vi "getValue.vi"(8 "error in (no error)":errorcluster, 11 "tBSONString in":refnum<class "tBSONString.lvclass">) -> (0 "error out":errorcluster, 2 "String":string, 3 "tBSONString out":refnum<class "tBSONString.lvclass">)   [LabVIEW 2013, in "BSON.lvlib" / "tBSONString.lvclass"]
uses:
  tBSONString.lvclass
  tBSONString.lvclass/tBSONString.ctl
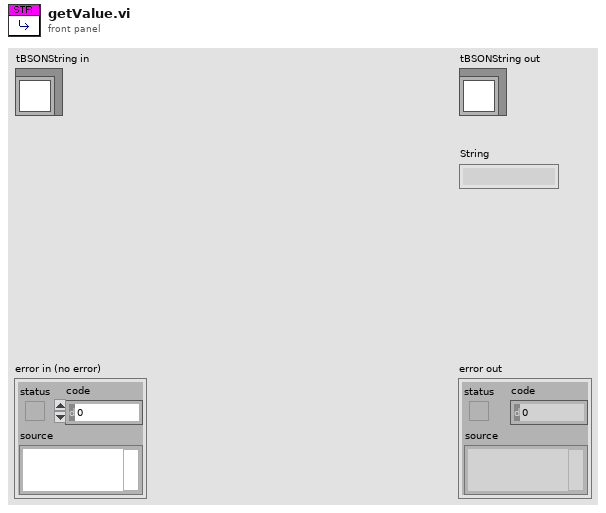
[diagram p1: front panel]
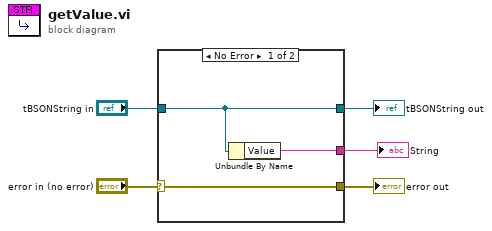
[diagram p0: block diagram]
diagram:
  n1 = case shown="No Error" "error in (no error)" {
    selector: "error in (no error)" -> [w8 w10]
    tunnel: [w8 w10] -> w4
    tunnel: [w7 w9] -> w2
    tunnel: "tBSONString in" -> [w7 w9]
    tunnel: [w6 _] -> w1
    frame No Error {
      n2 = Unbundle By Name(w7) -> ("Value"=w6:string)
    }
    frame Error {
    }
  }
  "error out" <- w4
  "tBSONString out" <- w2
  "String" <- w1
